vi "Set Allowed Security Protocol.vi"(8 "error in (no error)":errorcluster, 11 "AllowedProtocols":i32[](array[ring]) items=["SystemDefault"=0, "Ssl3"=48, "Tls"=192, "Tls11"=768, "Tls12"=3072, "Tls13"=12288]) -> (0 "error out":errorcluster)   [LabVIEW 2018, in "HttpClient_NET.lvlib" / "HttpClient_NET.lvclass"]
doc: "<b> </b> <b> </b>\nHttpClient_NET\nJustin Young - Viviota\nCopyright (c) 2021\nLicense: BSD"
uses:
  HttpClient_NET.lvclass
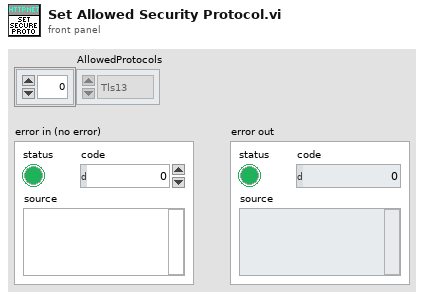
[diagram p1: front panel]
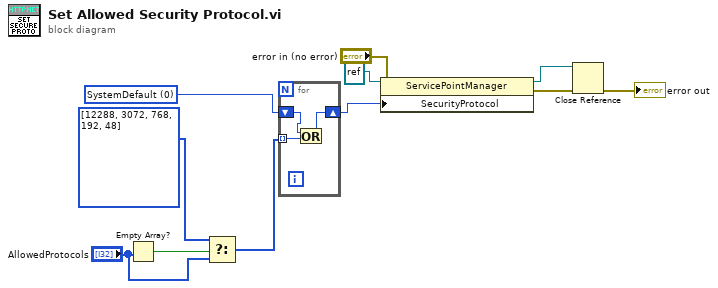
[diagram p0: block diagram]
diagram:
  w10 = 0 items=["SystemDefault"=0, "Ssl3"=48, "Tls"=192, "Tls11"=768, "Tls12"=3072, "Tls13"=12288] ("SecurityProtocol")
  w6 = i32[] [12288, 3072, 768, 192, 48] items=["SystemDefault"=0, "Ssl3"=48, "Tls"=192, "Tls11"=768, "Tls12"=3072, "Tls13"=12288]
  n1 = Empty Array?(array="AllowedProtocols") -> (empty?=w4:bool)
  n2 = Select(t=w6, s=w4, f="AllowedProtocols") -> (s? t:f=w3:i32[])
  n3 = for {
    tunnel: w3 -> [w14] mode=indexing
    shift-right: [w12] -> w11
    shift-left: w10 -> [w13]
    n4 = Or(x=w13, y=w14) -> (x .or. y?=w12:i32)
  }
  n5 = property class="ServicePointManager"(reference=refnum<k24> refnum, error in="error in (no error)", "SecurityProtocol"=w11) -> (reference out=w1:refnum<k24>, error out=w8:errorcluster)
  n6 = Close Reference(reference=w1, error in (no error)=w8) -> (error out=→"error out":errorcluster)
